vi "SMR_LabVIEW_V7.71.vi"() -> ()   [LabVIEW 2025]
uses:
  <vilib>/DAQmx/write.llb/DAQmx Write (Analog DBL 1Chan 1Samp).vi
  <vilib>/DAQmx/read.llb/DAQmx Read (Analog 1D DBL NChan 1Samp).vi
  <vilib>/DAQmx/read.llb/DAQmx Read (Analog 2D DBL NChan NSamp).vi
  <vilib>/Analysis/baseanly.llb/Mean (DBL).vi
  <vilib>/DAQmx/create/channels.llb/DAQmx Create Channel (AI-Temperature-Thermocouple).vi
  <vilib>/DAQmx/create/channels.llb/DAQmx Create Channel (AI-Voltage-Basic).vi
  <vilib>/DAQmx/create/channels.llb/DAQmx Create Channel (AO-Voltage-Basic).vi
  <vilib>/DAQmx/miscellaneous.llb/DAQmx Fill In Error Info.vi
  <vilib>/DAQmx/configure/timing.llb/DAQmx Timing (Sample Clock).vi
  <vilib>/addons/control/pid/pid.llb/PID (DBL).vi
  <vilib>/measure/maspectr.llb/FFT Power Spectrum and PSD for 1 Chan.vi
  <vilib>/measure/matone.llb/Extract Single Tone Information 1 Chan.vi
  <vilib>/addons/control/pid/NI_PID_pid.lvlib
  <vilib>/Analysis/NI_AALBase.lvlib
  <vilib>/ptbypt/NI_PtbyPt.lvlib
  <vilib>/measure/NI_MAPro.lvlib
panel:
  out "Time in Steady State (s)":dbl
  in  "Steady-State Dwell (s)":dbl
  out "Main Loop Flow (GPM)":dbl
  out "FM Amplitude":dbl
  out "FM Frequency":dbl
  out "Spectrum":cluster{"f0":dbl, "df":dbl, "magnitude":dbl[]}(graph)
  out "Raw Signal":waveform(dbl)(graph)
  out "Smoothed HX Flow (GPM)":dbl
  out "Flow History":dbl(graph)
  out "HX Flow (GPM)":dbl
  out "Voltage Across Rod (V)":dbl format="%0.2f"
  out "Current Run Folder":path
  in  "Log Root Folder":path=path "C:/Users/LocalUser/Documents/GitHub/thermal-loop/resources/v0.1.1/data/001"
  out "Raw NI9201 \nVoltage Display":T1
  in  "Loop Period (ms)":dbl=1000.0
  in  "Stop":bool
  out "Auto Steady State Threshold (deg C/min)":dbl
  out "Max dT/dt (deg C/min)":dbl
  out "Temp Change Rate (deg C/min)":dbl
  out "5-Min Baseline Complete":bool
  out "Rate Window Ready":bool
  out "Steady State":bool
  in  "Voltage Limit (V)":dbl=10.0
  in  "Temperature Limit (C)":dbl=50.0
  in  "Pressure Limit (psi)":dbl=15.0
  out "Max Voltage":bool
  out "Max Temperature":bool
  out "Max Pressure":bool
  out "Heat Exchanger Pressure History":dbl(graph)
  out "Main Loop Pressure History":T2(graph)
  out "Overall Avg Pressure (psi)":dbl
  out "Heat Exchanger Pressure P6 (psi)":dbl
  out "Main Loop Avg Pressure (psi)":dbl
  out "Pressure Display":T3
  out "Overall Pressure History":T4(graph)
  out "Max Loop Pressure (psi)":dbl
  out "Heat Exchanger Temperature History":cluster{"Waveform":dbl, "Waveform":dbl}(graph)
  out "Main Loop Temeperature History":T5(graph)
  out "Heat Exchanger Avg Temp (deg C)":dbl
  out "Temperature Display":T6
  out "Overall Temperature History":T7(graph)
  out "Overall Avg Temp (deg C)":dbl
  out "Max Loop Temp (deg C)":dbl
  out "Final P-Valve Voltage (V)":dbl
  out "PID Trim Voltage (V)":dbl
  in  "PID Temp Setpoint (deg C)":dbl
  in  "Auto PID Enable":bool
  in  "Manual P-Valve Voltage (V)":dbl min=0.0 max=10.0
  out "Main Loop Avg Temp (deg C)":dbl
  # "Heat Exchanger Flow"
  # "Control/Troubleshoot"
  # "Steady State"
  # "Emergency Indicators"
  # "Pressure"
  # "Temperature"
  # "Proportional Valve Control"
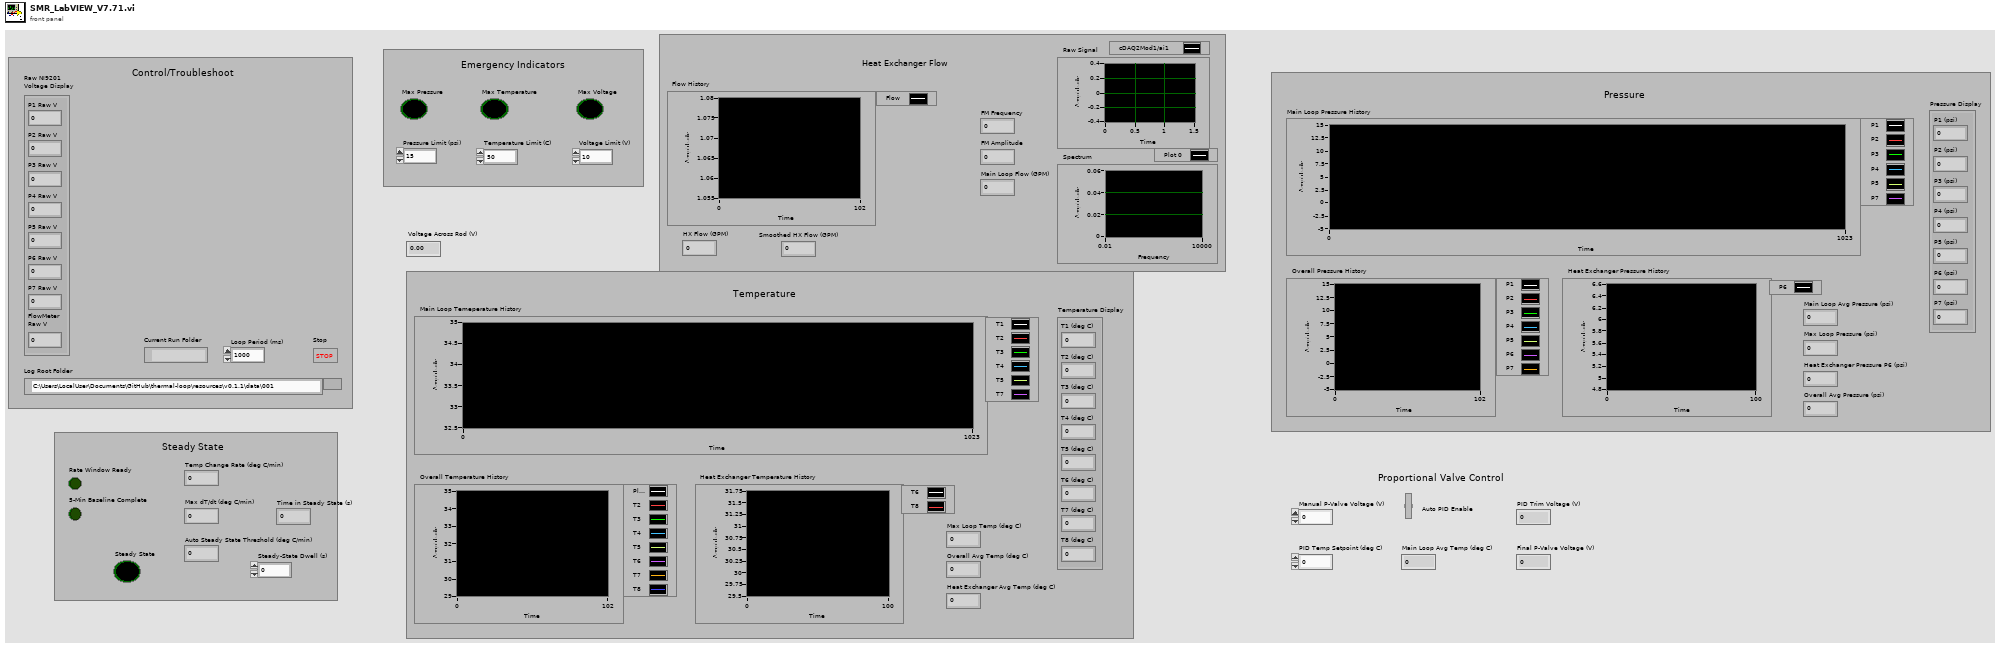
[diagram p1: front panel]
types:
  T1 = cluster{"P1 Raw V":dbl, "P2 Raw V":dbl, "P3 Raw V":dbl, "P4 Raw V":dbl, "P5 Raw V":dbl, "P6 Raw V":dbl, "P7 Raw V":dbl, "FlowMeter\nRaw V":dbl}
  T2 = cluster{"P1":dbl, "P2":dbl, "P3":dbl, "P4":dbl, "P5":dbl, "P7":dbl}
  T3 = cluster{"P1 (psi)":dbl, "P2 (psi)":dbl, "P3 (psi)":dbl, "P4 (psi)":dbl, "P5 (psi)":dbl, "P6 (psi)":dbl, "P7 (psi)":dbl}
  T4 = cluster{"P1":dbl, "P2":dbl, "P3":dbl, "P4":dbl, "P5":dbl, "P6":dbl, "P7":dbl}
  T5 = cluster{"Waveform":dbl, "Waveform":dbl, "Waveform":dbl, "Waveform":dbl, "Waveform":dbl, "Waveform":dbl}
  T6 = cluster{"T1 (deg C)":dbl, "T2 (deg C)":dbl, "T3 (deg C)":dbl, "T4 (deg C)":dbl, "T5 (deg C)":dbl, "T6 (deg C)":dbl, "T7 (deg C)":dbl, "T8 (deg C)":dbl}
  T7 = cluster{"Waveform":dbl, "Waveform":dbl, "Waveform":dbl, "Waveform":dbl, "Waveform":dbl, "Waveform":dbl, "Waveform":dbl, "Waveform":dbl}
  T8 = enum16{"open", "replace", "create", "open or create", "replace or create", "replace or create with confirmation"}
  T9 = cluster{"proportional gain (Kc)":dbl, "integral time (Ti, min)":dbl, "derivative time (Td, min)":dbl}
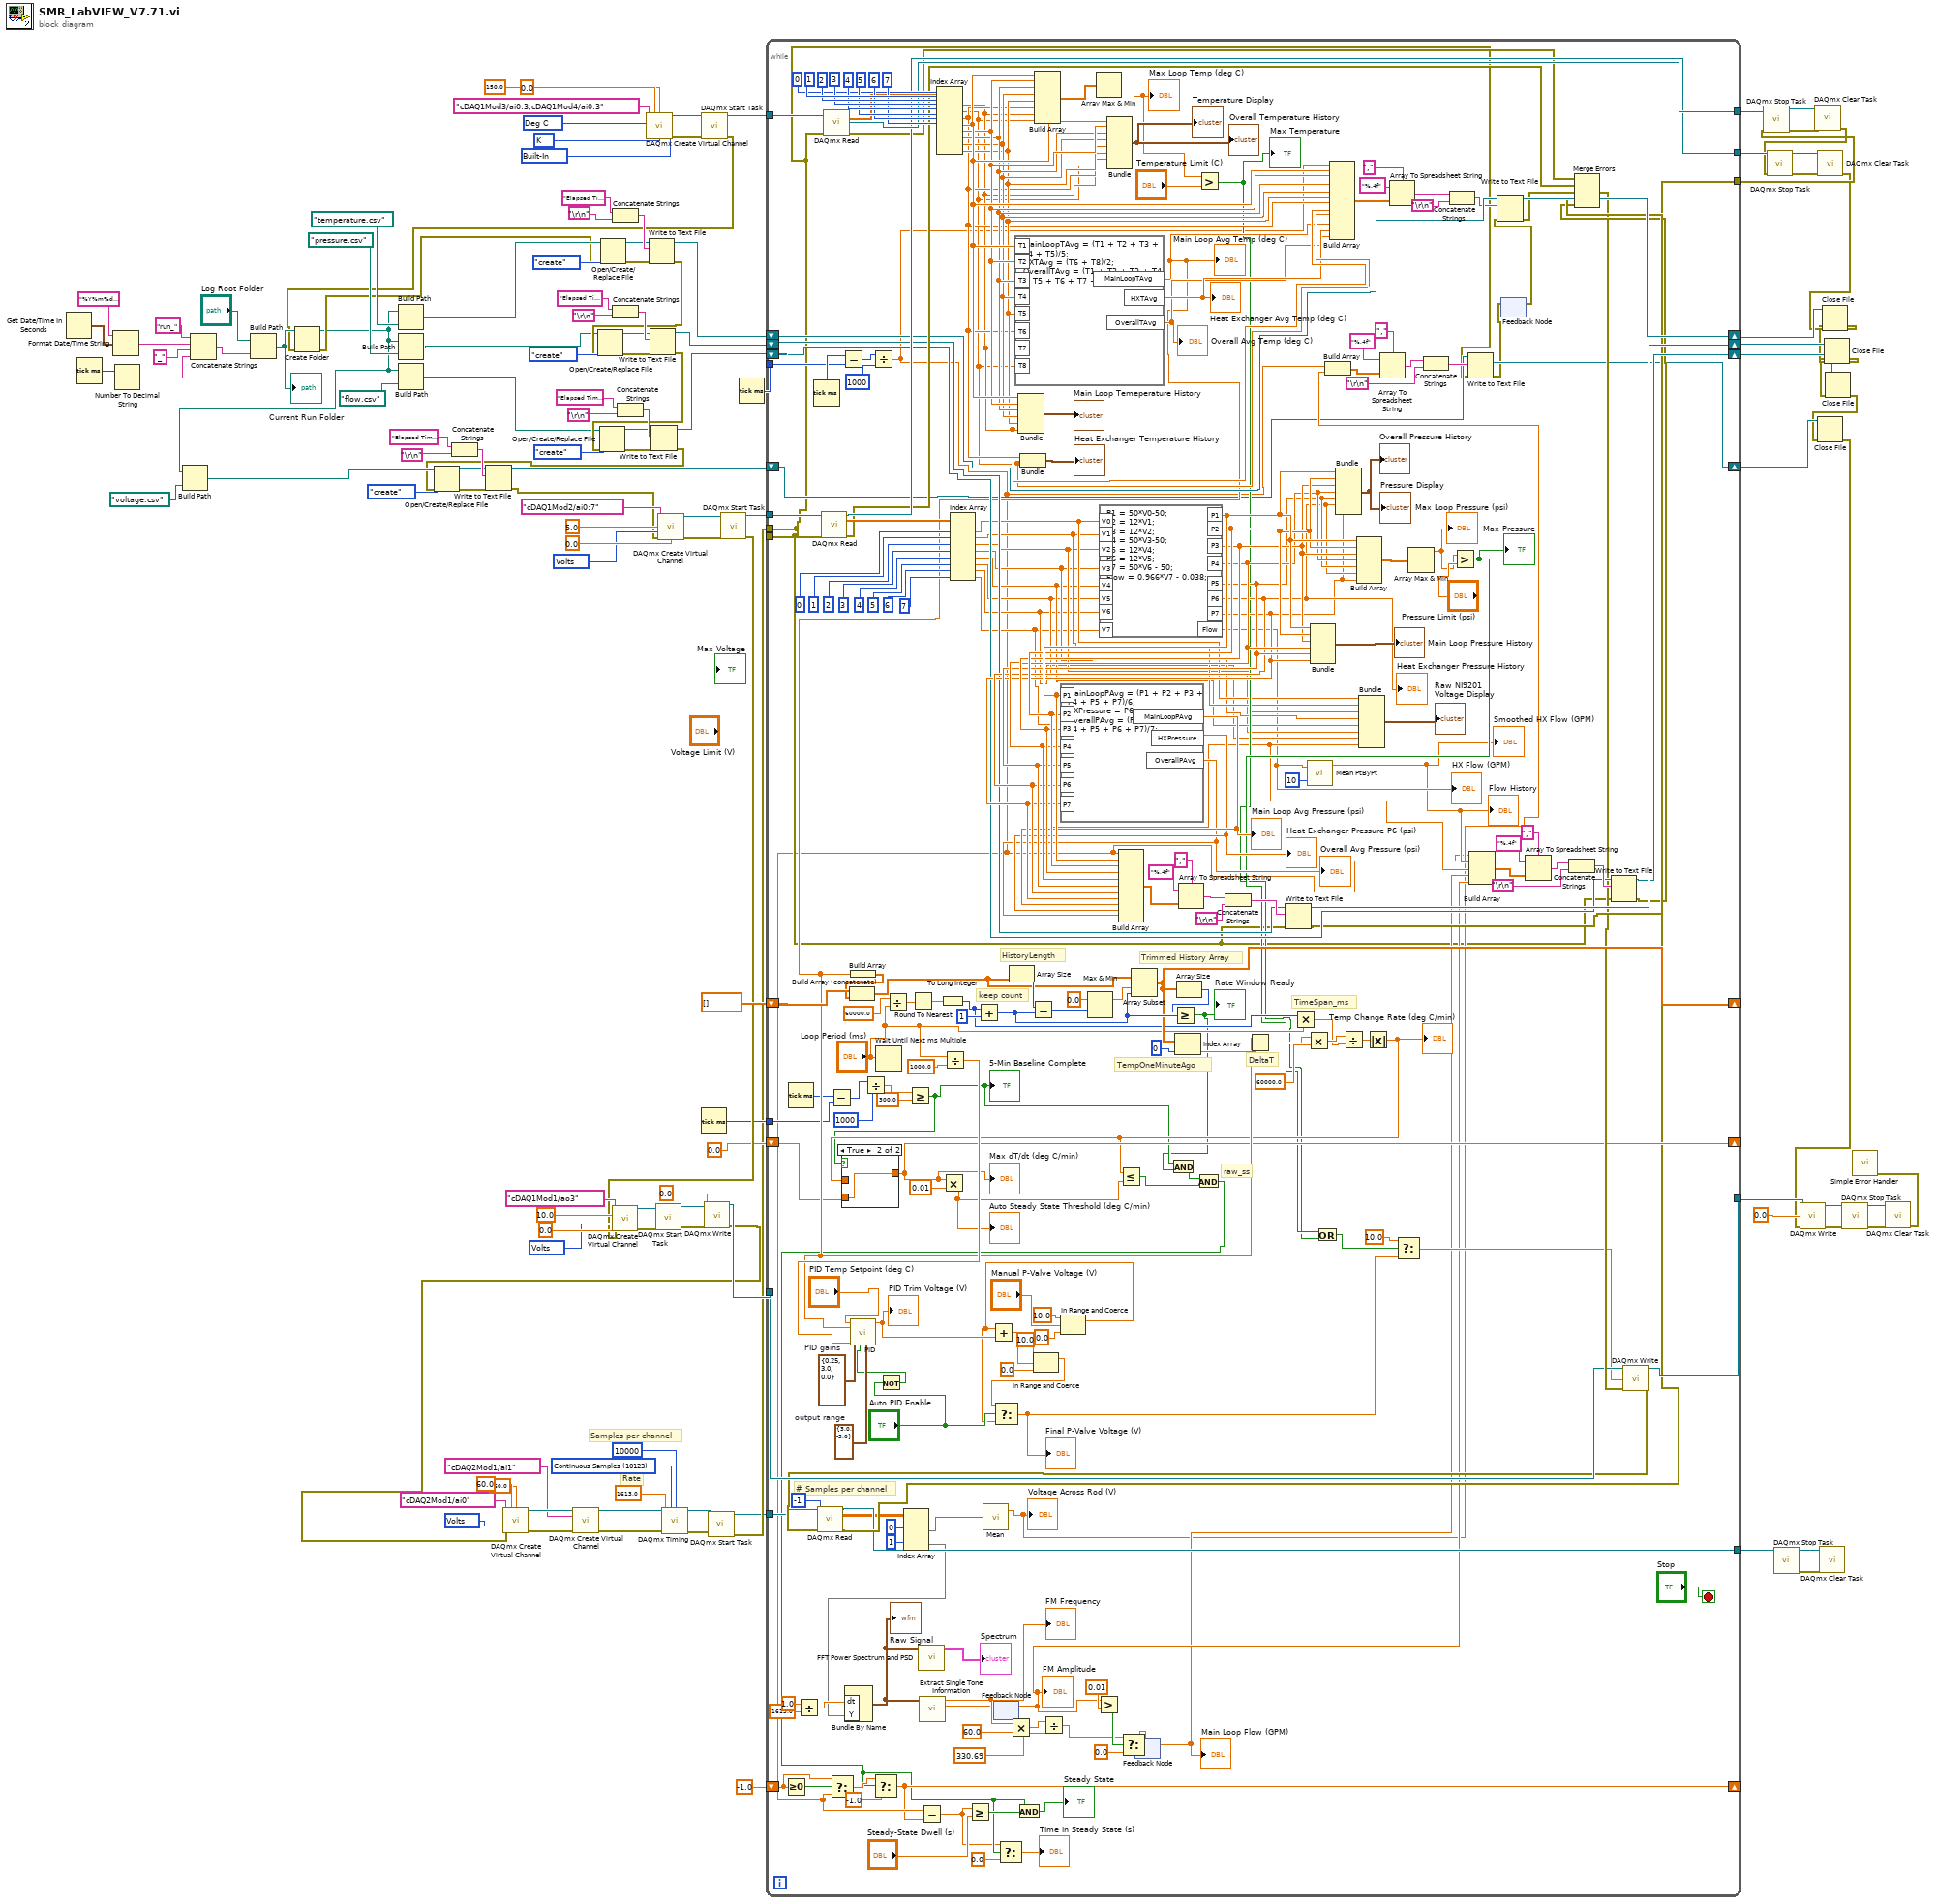
[diagram p0: block diagram]
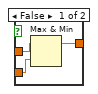
[diagram p2: hidden frame]
diagram:
  w31 = 10123 items=["Finite Samples"=10178, "Continuous Samples"=10123, "Hardware Timed Single Point"=12522] ("sample mode")
  w33 = 10348 items=["Volts"=10348, "From Custom Scale"=10065] ("units")
  w53 = 10348 items=["Volts"=10348, "From Custom Scale"=10065] ("units")
  w117 = 10200 items=["Built-In"=10200, "Constant Value"=10116, "Channel"=10113] ("cjc source")
  w118 = 10073 items=["J"=10072, "K"=10073, "N"=10077, "R"=10082, "S"=10085, "T"=10086, "B"=10047, "E"=10055] ("thermocouple type")
  w119 = 10143 items=["Deg C"=10143, "Deg F"=10144, "Kelvins"=10325, "Deg R"=10145, "From Custom Scale"=10065] ("units")
  w126 = 10348 items=["Volts"=10348, "From Custom Scale"=10065] ("units")
  # "Samples per channel"
  # "Rate"
  n1 = Get Date/Time In Seconds() -> (seconds since 1Jan1904=w75:timestamp)
  n2 = Tick Count (ms)() -> (millisecond timer value=w73:u32)
  n3 = Format Date/Time String(time format string (%c)="%Y%m%d_%H%M%S", seconds (now)=w75) -> (date/time string=w70:string)  [unwired: 1 in]
  n4 = Number To Decimal String(number=w73) -> (decimal integer string=w71:string)  [unwired: 1 in]
  n5 = Concatenate Strings("run_" ("string"), w70, "_" ("string"), w71) -> (w67:string)
  n6 = Build Path(base path="Log Root Folder", name or relative path=w67) -> (appended path=w66:path)
  "Current Run Folder" <- w66
  n7 = Concatenate Strings("Elapsed Time (s), Rod voltage (V)", "\r\n") -> (w15:string)
  n8 = Concatenate Strings("Elapsed Time (s),T1 (deg C),T2 (deg C),T3 (deg C),T4 (deg C),T5 (deg C),T6 (deg C),T7 (deg C),T8 (deg C),Main Loop Avg Temp (deg C),HX Avg Temp (deg C),Overall Avg Temp (deg C)", "\r\n") -> (w100:string)
  n9 = Concatenate Strings("Elapsed Time (s),P1 (psi),P2 (psi),P3 (psi),P4 (psi),P5 (psi),P6 (psi),P7 (psi),Main Loop Avg Pressure (psi),HX Pressure (psi),Overall Avg Pressure (psi)", "\r\n") -> (w98:string)
  n10 = Concatenate Strings("Elapsed Time (s),Heat Exchanger Flow (GPM),Flow Raw Voltage (V), Main Loop Flow (GPM), Flow Signal Amplitude (V)", "\r\n") -> (w94:string)
  n11 = call-poly <vilib>:"DAQmx Create Virtual Channel.vi"("maximum value"=150.0, "minimum value"=0.0, "physical channels"=tag "cDAQ1Mod3/ai0:3,cDAQ1Mod4/ai0:3", "cjc source"=w117, "units"=w119, "thermocouple type"=w118) -> ("task out"=w116:refnum<k21>, "error out"=w115:errorcluster)  [unwired: 8 in]
  n12 = Tick Count (ms)() -> (millisecond timer value=w38:u32)
  n13 = call <vilib>:"DAQmx Start Task.vi"("task/channels in"=w116, "error in"=w115) -> ("task out"=w114:refnum<k21>, "error out"=w59:errorcluster)  [unwired: 12 in]
  n14 = Create Folder(path (use dialog)=w66, error in=w59) -> (created path=w9:path, error out=w58:errorcluster)  [unwired: 1 in, 1 out]
  n15 = Build Path(base path=w9, name or relative path=path "voltage.csv") -> (appended path=w10:path)
  n16 = Build Path(base path=w9, name or relative path=path "temperature.csv") -> (appended path=w65:path)
  n17 = Build Path(base path=w9, name or relative path=path "pressure.csv") -> (appended path=w64:path)
  n18 = Build Path(base path=w9, name or relative path=path "flow.csv") -> (appended path=w63:path)
  n19 = Open/Create/Replace File(file path (use dialog)=w65, error in=w58, operation (0:open)=T8."create") -> (refnum out=w99:refnum<file>, error out=w83:errorcluster)  [unwired: 3 in, 1 out]
  n20 = Write to Text File(file (use dialog)=w99, text=w100, error in=w83) -> (refnum out=w90:refnum<file>, error out=w82:errorcluster)  [unwired: 1 in, 1 out]
  n21 = Open/Create/Replace File(file path (use dialog)=w64, error in=w82, operation (0:open)=T8."create") -> (refnum out=w97:refnum<file>, error out=w81:errorcluster)  [unwired: 3 in, 1 out]
  n22 = Write to Text File(file (use dialog)=w97, text=w98, error in=w81) -> (refnum out=w89:refnum<file>, error out=w80:errorcluster)  [unwired: 1 in, 1 out]
  n23 = Open/Create/Replace File(file path (use dialog)=w63, error in=w80, operation (0:open)=T8."create") -> (refnum out=w93:refnum<file>, error out=w79:errorcluster)  [unwired: 3 in, 1 out]
  n24 = Write to Text File(file (use dialog)=w93, text=w94, error in=w79) -> (refnum out=w88:refnum<file>, error out=w7:errorcluster)  [unwired: 1 in, 1 out]
  n25 = Open/Create/Replace File(file path (use dialog)=w10, error in=w7, operation (0:open)=T8."create") -> (refnum out=w14:refnum<file>, error out=w11:errorcluster)  [unwired: 3 in, 1 out]
  n26 = Write to Text File(file (use dialog)=w14, text=w15, error in=w11) -> (refnum out=w5:refnum<file>, error out=w6:errorcluster)  [unwired: 1 in, 1 out]
  n27 = call-poly <vilib>:"DAQmx Create Virtual Channel.vi"("maximum value"=5.0, "minimum value"=0.0, "physical channels"=tag "cDAQ1Mod2/ai0:7", "units"=w126, "error in"=w6) -> ("task out"=w125:refnum<k21>, "error out"=w124:errorcluster)  [unwired: 9 in]
  n28 = call <vilib>:"DAQmx Start Task.vi"("task/channels in"=w125, "error in"=w124) -> ("task out"=w123:refnum<k21>, "error out"=w46:errorcluster)  [unwired: 12 in]
  n29 = call-poly <vilib>:"DAQmx Create Virtual Channel.vi"("maximum value"=10.0, "minimum value"=0.0, "physical channels"=tag "cDAQ1Mod1/ao3", "units"=w53, "error in"=w46) -> ("task out"=w52:refnum<k21>, "error out"=w51:errorcluster)  [unwired: 9 in]
  n30 = call <vilib>:"DAQmx Start Task.vi"("task/channels in"=w52, "error in"=w51) -> ("task out"=w50:refnum<k21>, "error out"=w49:errorcluster)  [unwired: 12 in]
  n31 = call-poly <vilib>:"DAQmx Write.vi"("task/channels in"=w50, "data"=0.0, "error in"=w49) -> ("task out"=w47:refnum<k21>, "error out"=w25:errorcluster)  [unwired: 10 in, 1 out]
  n32 = call-poly <vilib>:"DAQmx Create Virtual Channel.vi"("maximum value"=60.0, "minimum value"=-60.0, "physical channels"=tag "cDAQ2Mod1/ai0", "units"=w33, "error in"=w25) -> ("task out"=w21:refnum<k21>, "error out"=w20:errorcluster)  [unwired: 9 in]
  n33 = call-poly <vilib>:"DAQmx Create Virtual Channel.vi"("task in"=w21, "physical channels"=tag "cDAQ2Mod1/ai1", "error in"=w20) -> ("task out"=w19:refnum<k21>, "error out"=w18:errorcluster)  [unwired: 11 in]
  n34 = call-poly <vilib>:"DAQmx Timing.vi"("task/channels in"=w19, "sample mode"=w31, "samples per channel"=10000, "rate"=1613.0, "error in"=w18) -> ("task out"=w29:refnum<k21>, "error out"=w28:errorcluster)  [unwired: 9 in]
  n35 = call <vilib>:"DAQmx Start Task.vi"("task/channels in"=w29, "error in"=w28) -> ("task out"=w23:refnum<k21>, "error out"=w24:errorcluster)  [unwired: 12 in]
  n36 = Tick Count (ms)() -> (millisecond timer value=w87:u32)
  n37 = while {
    tunnel: w123 -> [w342]
    tunnel: w114 -> [w325]
    tunnel: [w315] -> w113
    tunnel: [w145] -> _
    tunnel: [w314] -> w112
    tunnel: [w190] -> w111
    shift-right: [w291] -> w86
    shift-left: w90 -> [w292]
    shift-right: [w272] -> w85
    shift-left: w89 -> [w273]
    shift-right: [w264] -> w84
    shift-left: w88 -> [w265]
    tunnel: w87 -> [w310]
    shift-right: [w243] -> _
    shift-left: dbl[] [] -> [w256]
    tunnel: w47 -> [w224]
    tunnel: w24 -> [w145]
    tunnel: [w231] -> w44
    tunnel: w38 -> [w213]
    shift-right: [w206] -> _
    shift-left: 0.0 -> [w208]
    tunnel: w23 -> [w189]
    tunnel: [w188] -> w22
    shift-right: [w146] -> w4
    shift-left: w5 -> [w147]
    shift-right: [w137] -> _
    shift-left: -1.0 -> [w141]
    stop <- "Stop" stop-if-true
    w229 = cluster{"output high":dbl, "output low":dbl} {"output high"=3.0, "output low"=-3.0}  # output range
    w230 = T9 {"proportional gain (Kc)"=0.25, "integral time (Ti, min)"=3.0, "derivative time (Td, min)"=0.0}  # PID gains
    # "raw_ss"
    # "# Samples per channel"
    # "TimeSpan_ms"
    # "DeltaT"
    # "TempOneMinuteAgo"
    # "Trimmed History Array"
    # "HistoryLength"
    # "keep count"
    n38 = Greater Or Equal To 0?(x=w141) -> (x >= 0?=w142:bool)
    n39 = Tick Count (ms)() -> (millisecond timer value=w214:u32)
    n40 = Divide(x=1.0, y=1613.0) -> (x/y=w161:dbl)
    n41 = Tick Count (ms)() -> (millisecond timer value=w311:u32)
    n42 = call-poly <vilib>:"DAQmx Read.vi"("task/channels in"=w342, "error in"=w145) -> ("task out"=w314:refnum<k21>, "data"=w333:dbl[], "error out"=w312:errorcluster)  [unwired: 11 in]
    n43 = call-poly <vilib>:"DAQmx Read.vi"("task/channels in"=w325, "error in"=w145) -> ("task out"=w315:refnum<k21>, "data"=w316:dbl[], "error out"=w313:errorcluster)  [unwired: 11 in]
    n44 = Subtract(x=w214, y=w213) -> (x-y=w212:u32)
    n45 = Subtract(x=w311, y=w310) -> (x-y=w309:u32)
    n46 = Divide(x=w212, y=u32 1000) -> (x/y=w210:dbl)
    n47 = Divide(x=w309, y=u32 1000) -> (x/y=w138:dbl)
    n48 = Select(t=w141, s=w142, f=w138) -> (s? t:f=w140:dbl)
    n49 = Wait Until Next ms Multiple(millisecond multiple="Loop Period (ms)") -> ()  [unwired: 1 out]
    n50 = Not(x="Auto PID Enable") -> (.not. x?=w225:bool)
    n51 = Divide(x=60000.0, y="Loop Period (ms)") -> (x/y=w253:dbl)
    n52 = Greater Or Equal?(x=w210, y=300.0) -> (x >= y?=w203:bool)
    "5-Min Baseline Complete" <- w203
    n53 = Round To Nearest(number=w253) -> (nearest integer value=w252:dbl)
    n54 = Index Array(array=w316, index #1=0 ("index"), index #2=1 ("index"), index #3=2 ("index"), index #4=3 ("index"), index #5=4 ("index"), index #6=5 ("index"), index #7=6 ("index"), index #8=7 ("index")) -> (element #1=w301:dbl, element #2=w300:dbl, element #3=w302:dbl, element #4=w307:dbl, element #5=w306:dbl, element #6=w305:dbl, element #7=w304:dbl, element #8=w303:dbl)
    n55 = To Long Integer(number=w252) -> (32bit integer=w240:i32)
    n56 = Divide(x="Loop Period (ms)", y=1000.0) -> (x/y=w226:dbl)
    n57 = Index Array(array=w333, index #1=0 ("index"), index #2=1 ("index"), index #3=2 ("index"), index #4=3 ("index"), index #5=4 ("index"), index #6=5 ("index"), index #7=6 ("index"), index #8=7 ("index")) -> (element #1=w187:dbl, element #2=w186:dbl, element #3=w185:dbl, element #4=w184:dbl, element #5=w183:dbl, element #6=w182:dbl, element #7=w181:dbl, element #8=w180:dbl)
    n58 = Add(x=w240, y=1) -> (x+y=w245:i32)
    n59 = feedback #1() -> (w157:dbl)  [unwired: 1 in]
    "FM Amplitude" <- w157
    n60 = formula code="MainLoopTAvg = (T1 + T2 + T3 + T4 + T5)/5;\nHXTAvg = (T6 + T8)/2;\nOverallTAvg = (T1 + T2 + T3 + T4 + T5 + T6 + T7 + T8)/8;"("T1"=w307, "T2"=w306, "T3"=w305, "T4"=w304, "T5"=w303, "T6"=w302, "T7"=w301, "T8"=w300) -> ("MainLoopTAvg"=w216:dbl, "HXTAvg"=w299:dbl, "OverallTAvg"=w298:dbl)
    "Overall Avg Temp (deg C)" <- w298
    "Main Loop Avg Temp (deg C)" <- w216
    "Heat Exchanger Avg Temp (deg C)" <- w299
    n61 = Build Array(w216) -> (w255:dbl[])
    n62 = Build Array (concatenate)(w256, w255) -> (w247:dbl[])
    n63 = call-poly <vilib>:"PID.vi"("reinitialize? (F)"=w225, "output range"=w229, "dt (s)"=w226, "PID gains"=w230, "process variable"=w216, "setpoint"="PID Temp Setpoint (deg C)") -> ("output"=w223:dbl)  [unwired: 4 in, 1 out]
    "PID Trim Voltage (V)" <- w223
    n64 = Array Size(array=w247) -> (size(s)=w250:i32)
    n65 = Bundle("Waveform"=w307, "Waveform"=w306, "Waveform"=w305, "Waveform"=w304, "Waveform"=w303, "Waveform"=w301) -> (→"Main Loop Temeperature History":T5)  [unwired: 1 in]
    n66 = Bundle("Waveform"=w302, "Waveform"=w300) -> (→"Heat Exchanger Temperature History":cluster{"Waveform":dbl, "Waveform":dbl})  [unwired: 1 in]
    n67 = Subtract(x=w250, y=w245) -> (x-y=w248:i32)
    n68 = Build Array(w307, w306, w305, w304, w303, w302, w301, w300) -> (w343:dbl[])
    n69 = In Range and Coerce(upper limit=10.0, x="Manual P-Valve Voltage (V)", lower limit=0.0) -> (coerced(x)=w218:dbl)  [unwired: 1 out]
    n70 = Add(x=w218, y=w223) -> (x+y=w222:dbl)
    n71 = In Range and Coerce(upper limit=10.0, x=w222, lower limit=0.0) -> (coerced(x)=w217:dbl)  [unwired: 1 out]
    n72 = Select(t=w217, s="Auto PID Enable", f=w218) -> (s? t:f=w195:dbl)
    "Final P-Valve Voltage (V)" <- w195
    n73 = Max & Min(x=0.0, y=w248) -> (max(x,y)=w246:dbl)  [unwired: 1 out]
    n74 = Array Max & Min(array=w343) -> (max value=w258:dbl)  [unwired: 3 out]
    "Max Loop Temp (deg C)" <- w258
    n75 = Greater?(x=w157, y=0.01) -> (0:w165:bool)
    n76 = formula code="P1 = 50*V0-50;\nP2 = 12*V1;\nP3 = 12*V2;\nP4 = 50*V3-50;\nP5 = 12*V4;\nP6 = 12*V5; \nP7 = 50*V6 - 50;\nFlow = 0.966*V7 - 0.038;"("V0"=w187, "V1"=w186, "V2"=w185, "V3"=w184, "V4"=w183, "V5"=w182, "V6"=w181, "V7"=w180) -> ("P1"=w290:dbl, "P2"=w289:dbl, "P3"=w288:dbl, "P4"=w287:dbl, "P5"=w286:dbl, "P6"=w285:dbl, "P7"=w284:dbl, "Flow"=w179:dbl)
    "HX Flow (GPM)" <- w179
    "Heat Exchanger Pressure History" <- w285
    n77 = formula code="MainLoopPAvg = (P1 + P2 + P3 + P4 + P5 + P7)/6;\nHXPressure = P6;\nOverallPAvg = (P1 + P2 + P3 + P4 + P5 + P6 + P7)/7;"("P1"=w290, "P2"=w289, "P3"=w288, "P4"=w287, "P5"=w286, "P6"=w285, "P7"=w284) -> ("MainLoopPAvg"=w283:dbl, "HXPressure"=w282:dbl, "OverallPAvg"=w281:dbl)
    "Overall Avg Pressure (psi)" <- w281
    "Heat Exchanger Pressure P6 (psi)" <- w282
    "Main Loop Avg Pressure (psi)" <- w283
    n78 = Bundle("Waveform"=w307, "Waveform"=w306, "Waveform"=w305, "Waveform"=w304, "Waveform"=w303, "Waveform"=w302, "Waveform"=w301, "Waveform"=w300) -> (→"Overall Temperature History" →"Temperature Display":T7)  [unwired: 1 in]
    n79 = Build Array(w138, w290, w289, w288, w287, w286, w285, w284, w283, w282, w281) -> (w280:dbl[])
    n80 = Array Subset(array=w247, index=w246, length=w245) -> (w243:dbl[])
    n81 = feedback #2() -> (w155:dbl)  [unwired: 1 in]
    "Main Loop Flow (GPM)" <- w155
    n82 = Index Array(array=w243, index=0) -> (element=w241:dbl)
    n83 = Array Size(array=w243) -> (size(s)=w244:i32)
    n84 = Greater Or Equal?(x=w244, y=w245) -> (x >= y?=w202:bool)
    "Rate Window Ready" <- w202
    n85 = And(x=w203, y=w202) -> (x .and. y?=w201:bool)
    n86 = Array To Spreadsheet String(delimiter (Tab)=",", array=w280, 3:"%.4f" ("format string")) -> (spreadsheet string=w276:string)
    n87 = Greater?(x=w258, y="Temperature Limit (C)") -> (0:w198:bool)
    "Max Temperature" <- w198
    n88 = Concatenate Strings(w276, "\r\n") -> (w274:string)
    n89 = Subtract(x=w216, y=w241) -> (x-y=w239:dbl)
    n90 = Write to Text File(file (use dialog)=w273, text=w274, error in=w145) -> (refnum out=w272:refnum<file>, error out=w262:errorcluster)  [unwired: 1 in, 1 out]
    n91 = Multiply(x=w240, y="Loop Period (ms)") -> (x*y=w236:dbl)
    n92 = Multiply(x=w239, y=60000.0) -> (x*y=w237:dbl)
    n93 = call <vilib>:"Mean PtByPt.vi"("x"=w179, "sample length"=10) -> ("mean"=w177:dbl)  [unwired: 2 in, 1 out]
    "Flow History" <- w177
    "Smoothed HX Flow (GPM)" <- w177
    n94 = Bundle("P1"=w290, "P2"=w289, "P3"=w288, "P4"=w287, "P5"=w286, "P7"=w284) -> (→"Main Loop Pressure History":T2)  [unwired: 1 in]
    n95 = Build Array(w138, w307, w306, w305, w304, w303, w302, w301, w300, w216, w299, w298) -> (w297:dbl[])
    n96 = Bundle("P1"=w290, "P2"=w289, "P3"=w288, "P4"=w287, "P5"=w286, "P6"=w285, "P7"=w284) -> (→"Overall Pressure History" →"Pressure Display":T4)  [unwired: 1 in]
    n97 = Divide(x=w237, y=w236) -> (x/y=w235:dbl)
    n98 = Build Array(w290, w289, w288, w287, w286, w285, w284) -> (w332:dbl[])
    n99 = Bundle("Waveform"=w187, "Waveform"=w186, "Waveform"=w185, "Waveform"=w184, "Waveform"=w183, "Waveform"=w182, "Waveform"=w181, "Waveform"=w180) -> (→"Raw NI9201 \nVoltage Display":T7)  [unwired: 1 in]
    n100 = Absolute Value(x=w235) -> (abs(x)=w205:dbl)
    "Temp Change Rate (deg C/min)" <- w205
    n101 = case shown="True" w203 {
      tunnel: w208 -> [w347 w348]
      tunnel: w205 -> [w346 _]
      tunnel: [w345 w348] -> w206
      frame False {
        n102 = Max & Min(x=w346, y=w347) -> (max(x,y)=w345:dbl)  [unwired: 1 out]
      }
      frame True {
      }
    }
    "Max dT/dt (deg C/min)" <- w206
    n103 = Multiply(x=w206, y=0.01) -> (x*y=w204:dbl)
    "Auto Steady State Threshold (deg C/min)" <- w204
    n104 = Less Or Equal?(x=w205, y=w204) -> (x <= y?=w200:bool)
    n105 = And(x=w201, y=w200) -> (x .and. y?=w133:bool)
    n106 = Select(t=w140, s=w133, f=-1.0) -> (s? t:f=w137:dbl)
    n107 = Subtract(x=w138, y=w137) -> (x-y=w132:dbl)
    n108 = Greater Or Equal?(x=w132, y="Steady-State Dwell (s)") -> (x >= y?=w135:bool)
    n109 = Select(t=w132, s=w133, f=0.0) -> (s? t:f=→"Time in Steady State (s)":dbl)
    n110 = And(x=w133, y=w135) -> (x .and. y?=→"Steady State":bool)
    n111 = Array To Spreadsheet String(delimiter (Tab)=",", array=w297, 3:"%.4f" ("format string")) -> (spreadsheet string=w294:string)
    n112 = Array Max & Min(array=w332) -> (max value=w259:dbl)  [unwired: 3 out]
    "Max Loop Pressure (psi)" <- w259
    n113 = Concatenate Strings(w294, "\r\n") -> (w277:string)
    n114 = Greater?(x=w259, y="Pressure Limit (psi)") -> (0:w199:bool)
    "Max Pressure" <- w199
    n115 = Or(x=w199, y=w198) -> (x .or. y?=w193:bool)
    n116 = Select(t=10.0, s=w193, f=w195) -> (s? t:f=w194:dbl)
    n117 = Build Array(w138, w177, w180, w155, w157) -> (w271:dbl[])
    n118 = feedback #3() -> (w143:errorcluster)  [unwired: 1 in]
    n119 = Write to Text File(file (use dialog)=w292, text=w277, error in=w143) -> (refnum out=w291:refnum<file>, error out=w263:errorcluster)  [unwired: 1 in, 1 out]
    n120 = Array To Spreadsheet String(delimiter (Tab)=",", array=w271, 3:"%.4f" ("format string")) -> (spreadsheet string=w267:string)
    n121 = Concatenate Strings(w267, "\r\n") -> (w266:string)
    n122 = Write to Text File(file (use dialog)=w265, text=w266, error in=w145) -> (refnum out=w264:refnum<file>, error out=w261:errorcluster)  [unwired: 1 in, 1 out]
    n123 = Merge Errors(w313, w312, w263, w262, w261) -> (w232:errorcluster)
    n124 = call-poly <vilib>:"DAQmx Write.vi"("task/channels in"=w224, "data"=w194, "error in"=w232) -> ("task out"=w231:refnum<k21>, "error out"=w191:errorcluster)  [unwired: 10 in, 1 out]
    n125 = call-poly <vilib>:"DAQmx Read.vi"("task/channels in"=w189, "number of samples per channel"=-1, "error in"=w191) -> ("task out"=w188:refnum<k21>, "data"=w176:dbl[][], "error out"=w190:errorcluster)  [unwired: 10 in]
    n126 = Index Array(array=w176, index (row) #1=0 ("index (row)"), index (row) #2=1 ("index (row)")) -> (element #1=w175:dbl[], element #2=w160:dbl[])  [unwired: 2 in]
    n127 = Bundle By Name("dt"=w161, "Y"=w160) -> (w159:waveform(dbl))  [unwired: 1 in]
    "Raw Signal" <- w159
    n128 = call-poly <vilib>:"FFT Power Spectrum and PSD.vi"("time signal"=w159) -> ("Power Spectrum / PSD"=→"Spectrum":cluster{"f0":dbl, "df":dbl, "magnitude":dbl[]})  [unwired: 7 in, 3 out]
    n129 = call-poly <vilib>:"Extract Single Tone Information.vi"("time signal in"=w159) -> ("detected amplitude"=w158:dbl, "detected frequency"=w171:dbl)  [unwired: 5 in, 4 out]
    "FM Frequency" <- w171
    n130 = call-poly <vilib>:"Mean.vi"("X"=w175) -> ("mean"=w150:dbl)  [unwired: 1 out]
    "Voltage Across Rod (V)" <- w150
    n131 = feedback-in #1(w158) -> ()
    n132 = Multiply(x=w171, y=60.0) -> (x*y=w169:dbl)
    n133 = Divide(x=w169, y=330.69) -> (x/y=w164:dbl)
    n134 = Select(t=w164, s=w165, f=0.0) -> (s? t:f=w156:dbl)
    n135 = feedback-in #2(w156) -> ()
    n136 = Build Array(w138, w150) -> (w149:dbl[])
    n137 = Array To Spreadsheet String(delimiter (Tab)=",", array=w149, 3:"%.4f" ("format string")) -> (spreadsheet string=w153:string)
    n138 = Concatenate Strings(w153, "\r\n") -> (w148:string)
    n139 = Write to Text File(file (use dialog)=w147, text=w148, error in=w145) -> (refnum out=w146:refnum<file>, error out=w144:errorcluster)  [unwired: 1 in, 1 out]
    n140 = feedback-in #3(w144) -> ()
  }
  n141 = call <vilib>:"DAQmx Stop Task.vi"("task/channels in"=w113, "error in"=w111) -> ("task out"=w110:refnum<k21>, "error out"=w108:errorcluster)  [unwired: 12 in]
  n142 = call <vilib>:"DAQmx Stop Task.vi"("task/channels in"=w22) -> ("task out"=w27:refnum<k21>, "error out"=w26:errorcluster)  [unwired: 13 in]
  n143 = call <vilib>:"DAQmx Clear Task.vi"("task in"=w110, "error in"=w108) -> ("error out"=w107:errorcluster)  [unwired: 13 in]
  n144 = call <vilib>:"DAQmx Stop Task.vi"("task/channels in"=w112, "error in"=w107) -> ("task out"=w109:refnum<k21>, "error out"=w106:errorcluster)  [unwired: 12 in]
  n145 = call <vilib>:"DAQmx Clear Task.vi"("task in"=w109, "error in"=w106) -> ("error out"=w78:errorcluster)  [unwired: 13 in]
  n146 = call <vilib>:"DAQmx Clear Task.vi"("task in"=w27, "error in"=w26) -> ()  [unwired: 13 in, 1 out]
  n147 = Close File(refnum=w86, error in=w78) -> (error out=w77:errorcluster)  [unwired: 1 out]
  n148 = Close File(refnum=w85, error in=w77) -> (error out=w76:errorcluster)  [unwired: 1 out]
  n149 = Close File(refnum=w84, error in=w76) -> (error out=w3:errorcluster)  [unwired: 1 out]
  n150 = Close File(refnum=w4, error in=w3) -> (error out=w2:errorcluster)  [unwired: 1 out]
  n151 = call-poly <vilib>:"DAQmx Write.vi"("task/channels in"=w44, "data"=0.0, "error in"=w2) -> ("task out"=w43:refnum<k21>, "error out"=w41:errorcluster)  [unwired: 10 in, 1 out]
  n152 = call <vilib>:"DAQmx Stop Task.vi"("task/channels in"=w43, "error in"=w41) -> ("task out"=w42:refnum<k21>, "error out"=w40:errorcluster)  [unwired: 12 in]
  n153 = call <vilib>:"DAQmx Clear Task.vi"("task in"=w42, "error in"=w40) -> ("error out"=w39:errorcluster)  [unwired: 13 in]
  n154 = call <vilib>:"Simple Error Handler.vi"("error in (no error)"=w39) -> ()  [unwired: 4 in, 5 out]
